vi "CurrentCorrection.vi"(0 "ProbeStationControl in":refnum<class "ProbeStationControl.lvclass">, 1 "Action":T1(ring), 3 "Current IN":dbl[](array[numeric]), 4 "settling\ndelay":i32) -> (5 "Current OUT":dbl[](array[numeric]), 6 "ProbeStationControl out":refnum<class "ProbeStationControl.lvclass">, 7 "Compliance exceeded?":bool, 8 "Current Reference 100V":dbl[](array[numeric]), 9 "Current Reference 10V":dbl[](array[numeric]))   [LabVIEW 2013]
uses:
  InstrControl/ProbeStationControl/ProbeStationControl.lvclass
  general_VIs/globals/QC_MeasurementSetup.vi
  InstrControl/InstrumentSetup.vi
  InstrControl/SupplyControl/SupplyControl.lvclass
  InstrControl/Switching/Switching.lvclass
  InstrControl/InstrControl.lvclass
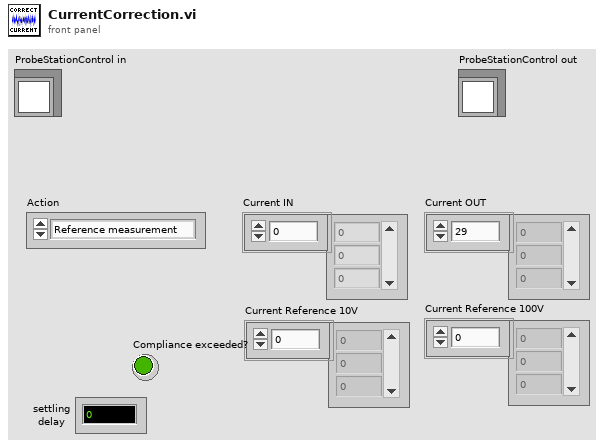
[diagram p1: front panel]
types:
  T1 = enum16{"Reference measurement", "Baseline correcetion 10V", "Baseline correcetion 100V", "Nothing"}
  T2 = cluster{"Bias Supply":refnum<class "SupplyControl.lvclass">, "SMU":refnum<class "SupplyControl.lvclass">, "LCR":refnum<class "LCRControl.lvclass">, "Probe Card Channels":i32, "Bias Voltage [V]":dbl, "First strip":i32, "Last strip":i32, "Base Voltage [V]":dbl, "Base Ramp Step [V]":dbl, "Base Ramp Interval [ms]":u32, "High Voltage [V]":dbl, "High Ramp Step [V]":dbl, "High Ramp Interval [ms]":u32, "Single Needle":bool, "ArduinoControl.lvclass":refnum<class "ArduinoControl.lvclass">, "Fraction of good strips [%]":dbl}
  T3 = cluster{"GPIB address":string, "Matrix address":string, "Mux1 address":string, "Mux2 address":string, "Matrix used?":bool, "Switching":refnum<class "Switching.lvclass">, "Matrix X Channels":cluster{"Bias Supply / SMU LO":i32, "Bias Supply / SMU HI":i32, "CV Box LO":i32, "CV Box HI":i32, "CV Box LO IN":i32, "CV Box HI IN":i32, "Volt meter LO":i32, "Volt meter HI":i32, "Mux1 C1":i32, "Mux1 C2":i32, "Mux2 C1":i32, "Mux2 C2":i32}}
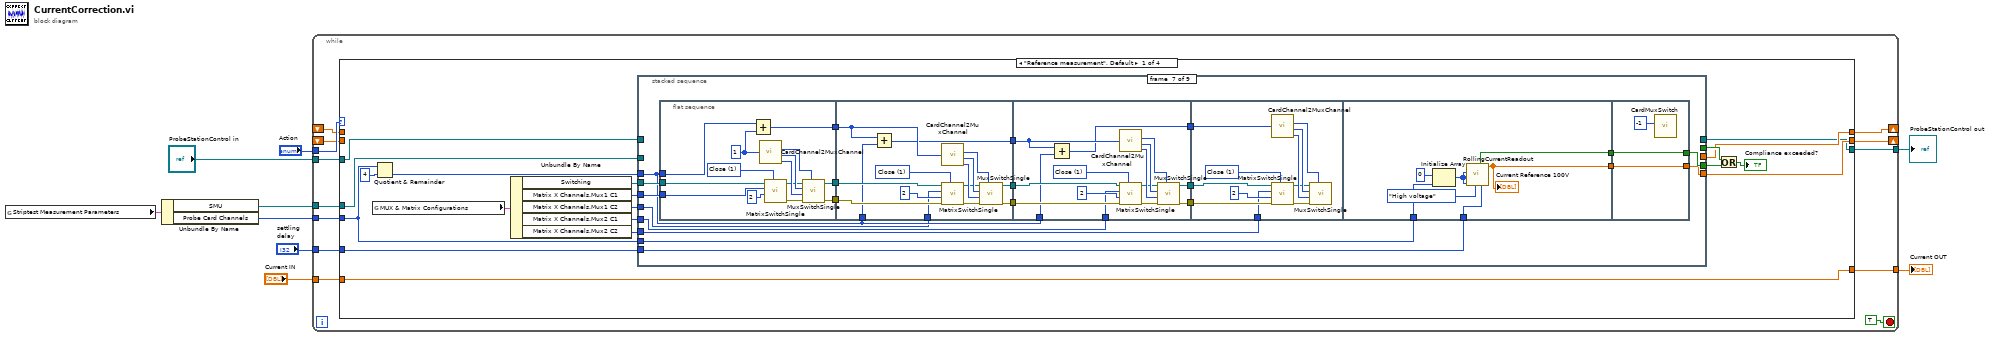
[diagram p0: block diagram]
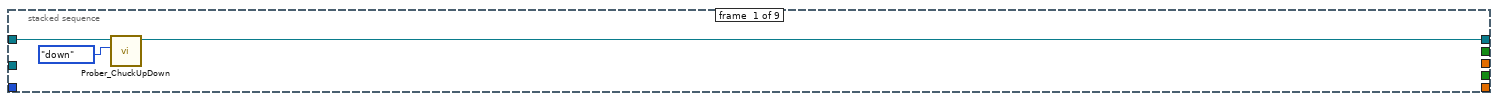
[diagram p2: hidden frame]
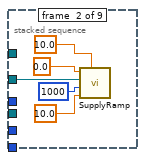
[diagram p3: hidden frame]
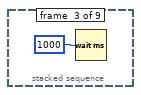
[diagram p4: hidden frame]
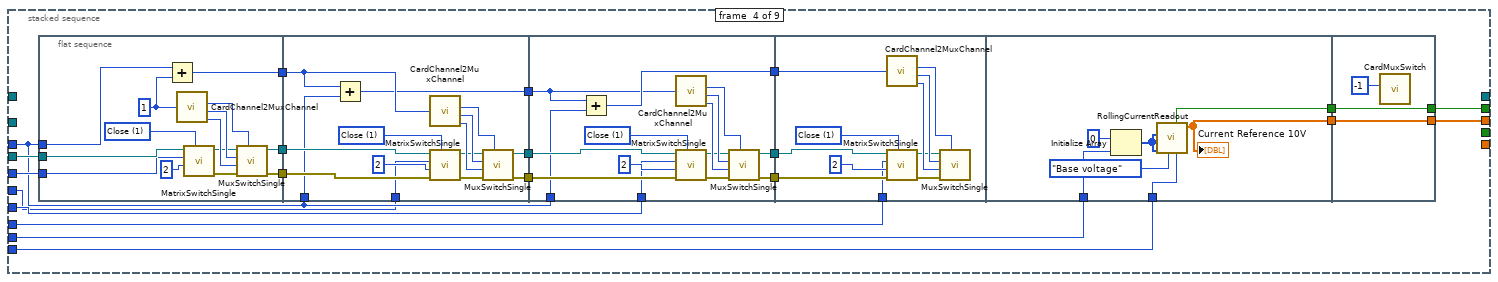
[diagram p5: hidden frame]
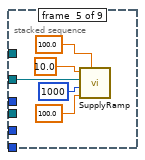
[diagram p6: hidden frame]
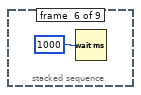
[diagram p7: hidden frame]
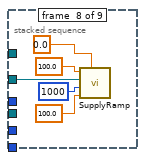
[diagram p8: hidden frame]
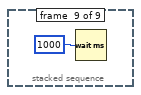
[diagram p9: hidden frame]
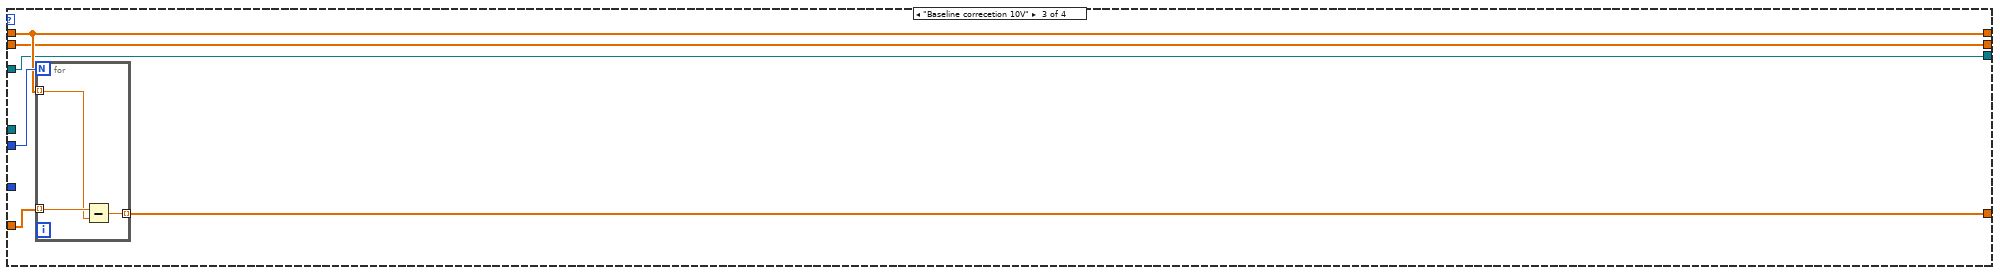
[diagram p11: hidden frame]
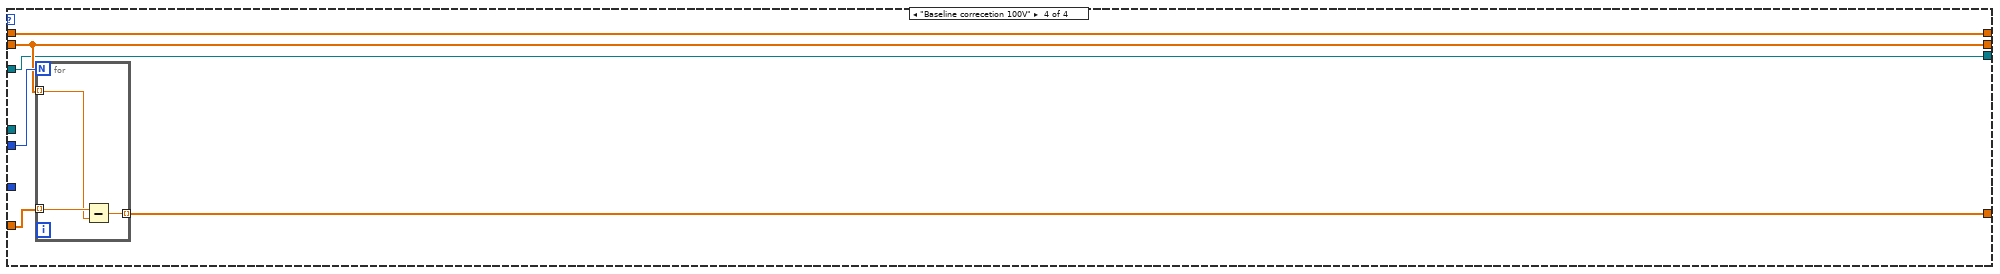
[diagram p12: hidden frame]
diagram:
  n1 = global read "QC_MeasurementSetup.vi" "Striptest Measurement Parameters"() -> (w3:T2)
  n2 = Unbundle By Name(w3) -> ("SMU"=w2:refnum<class "SupplyControl.lvclass">, "Probe Card Channels"=w1:i32)
  n3 = while {
    tunnel: "Action" -> [w22]
    tunnel: w1 -> [w21]
    tunnel: [w20] -> w8
    tunnel: "Current IN" -> [w19]
    shift-right: [w17] -> _
    shift-left: _ -> [w15]
    shift-right: [w16] -> _
    shift-left: _ -> [w14]
    tunnel: "settling\ndelay" -> [w13]
    tunnel: "ProbeStationControl in" -> [w12]
    tunnel: [w11] -> w4
    tunnel: w2 -> [w10]
    stop <- TRUE stop-if-true
    n4 = case shown="\"Reference measurement\", Default" w22 {
      tunnel: w21 -> [w24 _ w244 w252]
      tunnel: [w41 w238 w243 w251] -> w20
      tunnel: w19 -> [w41 w238 w242 w253]
      tunnel: [w37 w236 w241 w249] -> w17
      tunnel: [w36 w237 w240 w250] -> w16
      tunnel: w15 -> [_ w236 w241 w249]
      tunnel: w14 -> [_ w237 w240 w250]
      tunnel: w13 -> [w35 _ _ _]
      tunnel: w12 -> [w32 w235 w239 w248]
      tunnel: [w31 w235 w239 w248] -> w11
      tunnel: w10 -> [w26 _ _ _]
      frame "Reference measurement", Default {
        n5 = global read "InstrumentSetup.vi" "MUX & Matrix Configurations"() -> (w34:T3)
        n6 = Quotient & Remainder(x=w24, y=4) -> (floor(x/y)=w23:i32)  [unwired: 1 out]
        n7 = Unbundle By Name(w34) -> ("Switching"=w33:refnum<class "Switching.lvclass">, "Matrix X Channels.Mux1 C1"=w30:i32, "Matrix X Channels.Mux1 C2"=w29:i32, "Matrix X Channels.Mux2 C1"=w28:i32, "Matrix X Channels.Mux2 C2"=w27:i32)
        n8 = stacked-sequence {
          tunnel: w24 -> [_ _ _ w61 _ _ w151 _ _]
          tunnel: [_ _ _ w71 _ _ _ _ _] -> w39
          tunnel: [_ _ _ _ _ _ w163 _ _] -> w38
          tunnel: [_ _ _ w70 _ _ _ _ _] -> w37
          tunnel: [_ _ _ _ _ _ w162 _ _] -> w36
          tunnel: w35 -> [_ _ _ w62 _ _ w146 _ _]
          tunnel: w26 -> [_ w45 _ _ w137 _ _ w229 _]
          tunnel: w33 -> [_ _ _ w69 _ _ w161 _ _]
          tunnel: w32 -> [w43 _ _ _ _ _ _ _ _]
          tunnel: [w42 _ _ _ _ _ _ _ _] -> w31
          tunnel: w30 -> [_ _ _ w68 _ _ w160 _ _]
          tunnel: w29 -> [_ _ _ w51 _ _ w143 _ _]
          tunnel: w28 -> [_ _ _ w53 _ _ w144 _ _]
          tunnel: w27 -> [_ _ _ w52 _ _ w145 _ _]
          tunnel: w23 -> [_ _ _ w54 _ _ w149 _ _]
          frame #0 {
            n9 = call "Prober_ChuckUpDown.vi"("Direction"=enum16{"up", "down"}."down", "ProbeStationControl in"=w43) -> ("ProbeStationControl out"=w42:refnum<class "ProbeStationControl.lvclass">)  [unwired: 7 in, 2 out]
          }
          frame #1 {
            n10 = call "SupplyRamp.vi"("Requested Voltage"=10.0, "Step Size"=10.0, "Step Delay"=1000, "Supply IN"=w45, "Starting Voltage"=0.0) -> ()  [unwired: 3 in, 4 out]
          }
          frame #2 {
            n11 = Wait (ms)(milliseconds to wait=1000) -> ()  [unwired: 1 out]
          }
          frame #3 {
            n12 = flat-sequence {
              tunnel: w69 -> [w79]
              tunnel: [w77] -> w67
              tunnel: w68 -> [w78]
              tunnel: [w76] -> w58
              tunnel: w54 -> [w73]
              tunnel: [w72] -> w57
              tunnel: w67 -> [w93]
              tunnel: [w92] -> w66
              tunnel: [w91] -> w59
              tunnel: w58 -> [w90]
              tunnel: w57 -> [w89]
              tunnel: [w88] -> w56
              tunnel: w54 -> [w87]
              tunnel: w51 -> [w86]
              tunnel: w66 -> [w108]
              tunnel: [w107] -> w65
              tunnel: [w106] -> w60
              tunnel: w59 -> [w105]
              tunnel: w56 -> [w103]
              tunnel: [w104] -> w55
              tunnel: w54 -> [w102]
              tunnel: w53 -> [w101]
              tunnel: w65 -> [w119]
              tunnel: w60 -> [w118]
              tunnel: w55 -> [w117]
              tunnel: w52 -> [w116]
              tunnel: [w131] -> w64
              tunnel: [w130] -> w63
              tunnel: w62 -> [w128]
              tunnel: w61 -> [w127]
              tunnel: [w135] -> w71
              tunnel: w64 -> [w135]
              tunnel: [w134] -> w70
              tunnel: w63 -> [w134]
              frame #0 {
                w74 = 1
                w75 = u16 1 items=["Open", "Close"] ("Switch action")
                n13 = Add(x=w73, y=w74) -> (x+y=w72:i32)
                n14 = call "CardChannel2MuxChannel.vi"("Probecard Channel No."=w74) -> ("Mux No.:"=w83:u32, "C1 / C2"=w84:i32, "Channel"=w85:i32)  [unwired: 1 out]
                n15 = call "MatrixSwitchSingle.vi"("Switch action"=w75, "Matrix Y"=2, "Matrix X"=w78, "Switching in"=w79) -> ("error out"=w80:errorcluster, "Switching out"=w81:refnum<class "Switching.lvclass">)  [unwired: 5 in, 1 out]
                n16 = call "MuxSwitchSingle.vi"("MUX address"=w83, "error in (no error)"=w80, "Channel"=w85, "C1 / C2"=w84, "Switching in"=w81) -> ("error out"=w76:errorcluster, "Switching out"=w77:refnum<class "Switching.lvclass">)  [unwired: 4 in, 1 out]
              }
              frame #1 {
                w97 = u16 1 items=["Open", "Close"] ("Switch action")
                n17 = Add(x=w89, y=w87) -> (x+y=w88:i32)
                n18 = call "CardChannel2MuxChannel.vi"("Probecard Channel No."=w89) -> ("Mux No.:"=w98:u32, "C1 / C2"=w99:i32, "Channel"=w100:i32)  [unwired: 1 out]
                n19 = call "MatrixSwitchSingle.vi"("Switch action"=w97, "error in (no error)"=w90, "Matrix Y"=2, "Matrix X"=w86, "Switching in"=w93) -> ("error out"=w95:errorcluster, "Switching out"=w94:refnum<class "Switching.lvclass">)  [unwired: 4 in, 1 out]
                n20 = call "MuxSwitchSingle.vi"("MUX address"=w98, "error in (no error)"=w95, "Channel"=w100, "C1 / C2"=w99, "Switching in"=w94) -> ("error out"=w91:errorcluster, "Switching out"=w92:refnum<class "Switching.lvclass">)  [unwired: 4 in, 1 out]
              }
              frame #2 {
                w114 = u16 1 items=["Open", "Close"] ("Switch action")
                n21 = Add(x=w103, y=w102) -> (x+y=w104:i32)
                n22 = call "CardChannel2MuxChannel.vi"("Probecard Channel No."=w103) -> ("Mux No.:"=w113:u32, "C1 / C2"=w112:i32, "Channel"=w111:i32)  [unwired: 1 out]
                n23 = call "MatrixSwitchSingle.vi"("Switch action"=w114, "error in (no error)"=w105, "Matrix Y"=2, "Matrix X"=w101, "Switching in"=w108) -> ("error out"=w109:errorcluster, "Switching out"=w110:refnum<class "Switching.lvclass">)  [unwired: 4 in, 1 out]
                n24 = call "MuxSwitchSingle.vi"("MUX address"=w113, "error in (no error)"=w109, "Channel"=w111, "C1 / C2"=w112, "Switching in"=w110) -> ("error out"=w106:errorcluster, "Switching out"=w107:refnum<class "Switching.lvclass">)  [unwired: 4 in, 1 out]
              }
              frame #3 {
                w123 = u16 1 items=["Open", "Close"] ("Switch action")
                n25 = call "CardChannel2MuxChannel.vi"("Probecard Channel No."=w117) -> ("Mux No.:"=w124:u32, "C1 / C2"=w125:i32, "Channel"=w126:i32)  [unwired: 1 out]
                n26 = call "MatrixSwitchSingle.vi"("Switch action"=w123, "error in (no error)"=w118, "Matrix Y"=2, "Matrix X"=w116, "Switching in"=w119) -> ("error out"=w121:errorcluster, "Switching out"=w120:refnum<class "Switching.lvclass">)  [unwired: 4 in, 1 out]
                n27 = call "MuxSwitchSingle.vi"("MUX address"=w124, "error in (no error)"=w121, "Channel"=w126, "C1 / C2"=w125, "Switching in"=w120) -> ()  [unwired: 4 in, 3 out]
              }
              frame #4 {
                n28 = Initialize Array(0, w127) -> (w133:i32[])
                n29 = call "RollingCurrentReadout.vi"("settling\ndelay"=w128, "Base/High Voltage?"=enum16{"Base voltage", "High voltage"}."Base voltage", "disabled channels IN"=w133, "Flag IN"=w133, "Current Array IN [nA]"=w133) -> ("Current Array OUT [nA]"=w130:dbl[], "Compliance exceeded"=w131:bool)  [unwired: 3 in, 2 out]
                "Current Reference 10V" <- w130
              }
              frame #5 {
                n30 = call "CardMuxSwitch.vi"("Switch to channel"=-1) -> ()  [unwired: 10 in, 1 out]
              }
            }
          }
          frame #4 {
            n31 = call "SupplyRamp.vi"("Requested Voltage"=100.0, "Step Size"=100.0, "Step Delay"=1000, "Supply IN"=w137, "Starting Voltage"=10.0) -> ()  [unwired: 3 in, 4 out]
          }
          frame #5 {
            n32 = Wait (ms)(milliseconds to wait=1000) -> ()  [unwired: 1 out]
          }
          frame #6 {
            n33 = flat-sequence {
              tunnel: w161 -> [w170]
              tunnel: [w168] -> w159
              tunnel: w160 -> [w169]
              tunnel: [w167] -> w154
              tunnel: w149 -> [w165]
              tunnel: [w164] -> w150
              tunnel: w159 -> [w185]
              tunnel: [w183] -> w158
              tunnel: w154 -> [w184]
              tunnel: [w182] -> w153
              tunnel: w150 -> [w180]
              tunnel: w149 -> [w181]
              tunnel: [w179] -> w148
              tunnel: w143 -> [w178]
              tunnel: w158 -> [w200]
              tunnel: [w198] -> w157
              tunnel: w153 -> [w199]
              tunnel: [w197] -> w152
              tunnel: w149 -> [w196]
              tunnel: w148 -> [w195]
              tunnel: [w194] -> w147
              tunnel: w144 -> [w193]
              tunnel: w157 -> [w211]
              tunnel: w152 -> [w210]
              tunnel: w147 -> [w209]
              tunnel: w145 -> [w208]
              tunnel: [w223] -> w156
              tunnel: [w222] -> w155
              tunnel: w151 -> [w220]
              tunnel: w146 -> [w219]
              tunnel: [w227] -> w163
              tunnel: w156 -> [w227]
              tunnel: [w226] -> w162
              tunnel: w155 -> [w226]
              frame #0 {
                w166 = 1
                w177 = u16 1 items=["Open", "Close"] ("Switch action")
                n34 = Add(x=w165, y=w166) -> (x+y=w164:i32)
                n35 = call "CardChannel2MuxChannel.vi"("Probecard Channel No."=w166) -> ("Mux No.:"=w174:u32, "C1 / C2"=w175:i32, "Channel"=w176:i32)  [unwired: 1 out]
                n36 = call "MatrixSwitchSingle.vi"("Switch action"=w177, "Matrix Y"=2, "Matrix X"=w169, "Switching in"=w170) -> ("error out"=w171:errorcluster, "Switching out"=w172:refnum<class "Switching.lvclass">)  [unwired: 5 in, 1 out]
                n37 = call "MuxSwitchSingle.vi"("MUX address"=w174, "error in (no error)"=w171, "Channel"=w176, "C1 / C2"=w175, "Switching in"=w172) -> ("error out"=w167:errorcluster, "Switching out"=w168:refnum<class "Switching.lvclass">)  [unwired: 4 in, 1 out]
              }
              frame #1 {
                w189 = u16 1 items=["Open", "Close"] ("Switch action")
                n38 = Add(x=w180, y=w181) -> (x+y=w179:i32)
                n39 = call "CardChannel2MuxChannel.vi"("Probecard Channel No."=w180) -> ("Mux No.:"=w190:u32, "C1 / C2"=w191:i32, "Channel"=w192:i32)  [unwired: 1 out]
                n40 = call "MatrixSwitchSingle.vi"("Switch action"=w189, "error in (no error)"=w184, "Matrix Y"=2, "Matrix X"=w178, "Switching in"=w185) -> ("error out"=w186:errorcluster, "Switching out"=w187:refnum<class "Switching.lvclass">)  [unwired: 4 in, 1 out]
                n41 = call "MuxSwitchSingle.vi"("MUX address"=w190, "error in (no error)"=w186, "Channel"=w192, "C1 / C2"=w191, "Switching in"=w187) -> ("error out"=w182:errorcluster, "Switching out"=w183:refnum<class "Switching.lvclass">)  [unwired: 4 in, 1 out]
              }
              frame #2 {
                w206 = u16 1 items=["Open", "Close"] ("Switch action")
                n42 = Add(x=w195, y=w196) -> (x+y=w194:i32)
                n43 = call "CardChannel2MuxChannel.vi"("Probecard Channel No."=w195) -> ("Mux No.:"=w205:u32, "C1 / C2"=w204:i32, "Channel"=w203:i32)  [unwired: 1 out]
                n44 = call "MatrixSwitchSingle.vi"("Switch action"=w206, "error in (no error)"=w199, "Matrix Y"=2, "Matrix X"=w193, "Switching in"=w200) -> ("error out"=w201:errorcluster, "Switching out"=w202:refnum<class "Switching.lvclass">)  [unwired: 4 in, 1 out]
                n45 = call "MuxSwitchSingle.vi"("MUX address"=w205, "error in (no error)"=w201, "Channel"=w203, "C1 / C2"=w204, "Switching in"=w202) -> ("error out"=w197:errorcluster, "Switching out"=w198:refnum<class "Switching.lvclass">)  [unwired: 4 in, 1 out]
              }
              frame #3 {
                w215 = u16 1 items=["Open", "Close"] ("Switch action")
                n46 = call "CardChannel2MuxChannel.vi"("Probecard Channel No."=w209) -> ("Mux No.:"=w216:u32, "C1 / C2"=w217:i32, "Channel"=w218:i32)  [unwired: 1 out]
                n47 = call "MatrixSwitchSingle.vi"("Switch action"=w215, "error in (no error)"=w210, "Matrix Y"=2, "Matrix X"=w208, "Switching in"=w211) -> ("error out"=w212:errorcluster, "Switching out"=w213:refnum<class "Switching.lvclass">)  [unwired: 4 in, 1 out]
                n48 = call "MuxSwitchSingle.vi"("MUX address"=w216, "error in (no error)"=w212, "Channel"=w218, "C1 / C2"=w217, "Switching in"=w213) -> ()  [unwired: 4 in, 3 out]
              }
              frame #4 {
                n49 = Initialize Array(0, w220) -> (w225:i32[])
                n50 = call "RollingCurrentReadout.vi"("settling\ndelay"=w219, "Base/High Voltage?"=enum16{"Base voltage", "High voltage"}."High voltage", "disabled channels IN"=w225, "Flag IN"=w225, "Current Array IN [nA]"=w225) -> ("Current Array OUT [nA]"=w222:dbl[], "Compliance exceeded"=w223:bool)  [unwired: 3 in, 2 out]
                "Current Reference 100V" <- w222
              }
              frame #5 {
                n51 = call "CardMuxSwitch.vi"("Switch to channel"=-1) -> ()  [unwired: 10 in, 1 out]
              }
            }
          }
          frame #7 {
            n52 = call "SupplyRamp.vi"("Requested Voltage"=0.0, "Step Size"=100.0, "Step Delay"=1000, "Supply IN"=w229, "Starting Voltage"=100.0) -> ()  [unwired: 3 in, 4 out]
          }
          frame #8 {
            n53 = Wait (ms)(milliseconds to wait=1000) -> ()  [unwired: 1 out]
          }
        }
        n54 = Or(x=w39, y=w38) -> (x .or. y?=→"Compliance exceeded?":bool)
      }
      frame "Nothing" {
      }
      frame "Baseline correcetion 10V" {
        n55 = for {
          N: w244 -> [_]
          tunnel: w241 -> [w246] mode=indexing
          tunnel: w242 -> [w247] mode=indexing
          tunnel: [w245] -> w243 mode=indexing
          n56 = Subtract(x=w247, y=w246) -> (x-y=w245:dbl)
        }
      }
      frame "Baseline correcetion 100V" {
        n57 = for {
          N: w252 -> [_]
          tunnel: w253 -> [w256] mode=indexing
          tunnel: w250 -> [w255] mode=indexing
          tunnel: [w254] -> w251 mode=indexing
          n58 = Subtract(x=w256, y=w255) -> (x-y=w254:dbl)
        }
      }
    }
  }
  "Current OUT" <- w8
  "ProbeStationControl out" <- w4
